vi "Get Args from Line.vi"(0 "Data Line":string) -> (4 "Channel":string, 6 "Sample Number":string, 8 "Arg1":string, 10 "Arg2":string, 15 "Arg3":string)   [LabVIEW 2014]
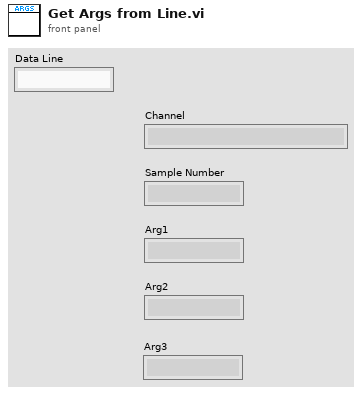
[diagram p1: front panel]
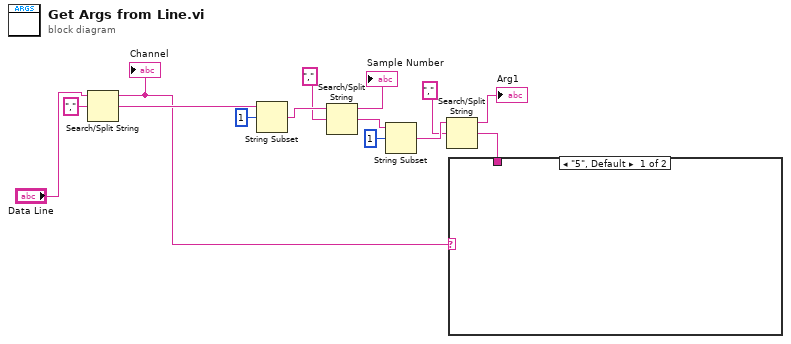
[diagram p0: block diagram]
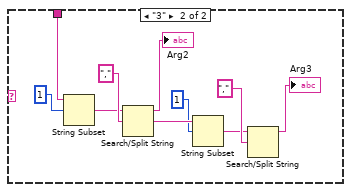
[diagram p2: hidden frame]
diagram:
  n1 = Search/Split String(string="Data Line", search string/char (-)=",") -> (substring before match=w1:string, match + rest of string=w4:string)  [unwired: 1 in, 1 out]
  "Channel" <- w1
  n2 = String Subset(string=w4, offset (0)=1) -> (substring=w7:string)  [unwired: 1 in]
  n3 = Search/Split String(string=w7, search string/char (-)=",") -> (substring before match=→"Sample Number":string, match + rest of string=w8:string)  [unwired: 1 in, 1 out]
  n4 = String Subset(string=w8, offset (0)=1) -> (substring=w11:string)  [unwired: 1 in]
  n5 = Search/Split String(string=w11, search string/char (-)=",") -> (substring before match=→"Arg1":string, match + rest of string=w14:string)  [unwired: 1 in, 1 out]
  n6 = case shown="\"5\", Default" w1 {
    tunnel: w14 -> [_ w15]
    frame "5", Default {
    }
    frame "3" {
      n7 = String Subset(string=w15, offset (0)=1) -> (substring=w17:string)  [unwired: 1 in]
      n8 = Search/Split String(string=w17, search string/char (-)=",") -> (substring before match=→"Arg2":string, match + rest of string=w21:string)  [unwired: 1 in, 1 out]
      n9 = String Subset(string=w21, offset (0)=1) -> (substring=w22:string)  [unwired: 1 in]
      n10 = Search/Split String(string=w22, search string/char (-)=",") -> (substring before match=→"Arg3":string)  [unwired: 1 in, 2 out]
    }
  }
